vi "sample1(BasicW).vi"() -> ()   [LabVIEW 2011]
panel:
  in  "OffsetTime":u32=20
  out "close_err":errorcluster caption="エラー出力" {"code" format="%04x"}
  out "write_err":errorcluster caption="エラー出力" {"code" format="%04x"}
  out "open_err":errorcluster {"code" format="%04x"}
  in  "ID":u8=1 max=253
  in  "Baudrate":u32=1000000
  in  "COM":refnum<visa-resource-name> caption="COMポート"
  in  "STOP":bool
  in  "POSITION":u16(knob) scale=0.0..4095.0
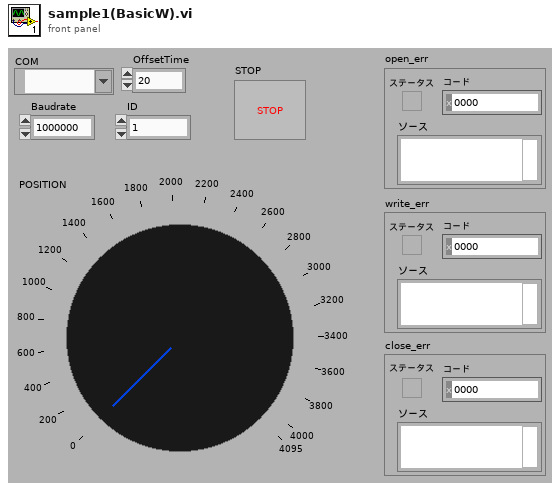
[diagram p1: front panel]
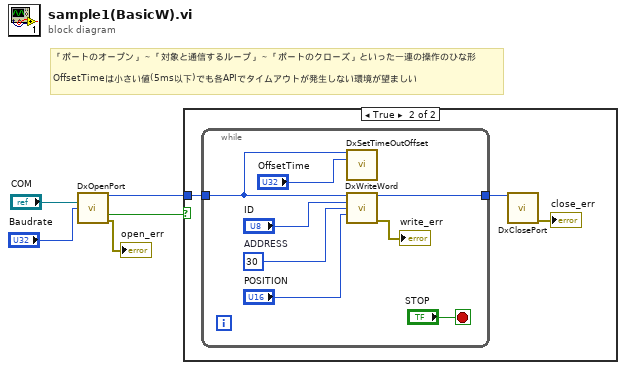
[diagram p0: block diagram]
diagram:
  # "「ポートのオープン」～「対象と通信するループ」～「ポートのクローズ」といった一連の操作のひな形\n\nOffsetTimeは小さい値(5ms以下)でも各APIでタイムアウトが発生しない環境が望ましい"
  n1 = call "DxOpenPort.vi"("port"="COM", "baudrate"="Baudrate") -> ("dvid"=w3:u32, "成功"=w1:bool, "エラー出力"=→"open_err":errorcluster)  [unwired: 11 in]
  n2 = case shown="TRUE" w1 {
    tunnel: w3 -> [_ w8]
    frame False {
    }
    frame True {
      n3 = while {
        tunnel: w8 -> [w10]
        tunnel: [w12] -> w7
        stop <- "STOP" stop-if-true
        w15 = u16 30  # ADDRESS
        n4 = call "DxSetTimeOutOffset.vi"("dvid in"=w10, "OffsetTime"="OffsetTime") -> ()  [unwired: 12 in, 2 out]
        n5 = call "DxWriteWord.vi"("dvid in"=w10, "id"="ID", "address"=w15, "data in"="POSITION") -> ("dvid out"=w12:u32, "エラー出力"=→"write_err":errorcluster)  [unwired: 9 in, 1 out]
      }
      n6 = call "DxClosePort.vi"("dvid"=w7) -> ("エラー出力"=→"close_err":errorcluster)  [unwired: 13 in, 1 out]
    }
  }
